vi "Split Numbers.vi"(0 "(hi.lo)":u16) -> (1 "low":u8, 2 "hi":u8)   [LabVIEW 2010]
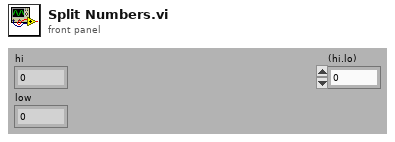
[diagram p1: front panel]
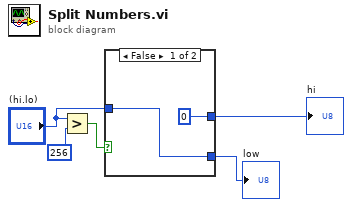
[diagram p0: block diagram]
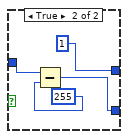
[diagram p2: hidden frame]
diagram:
  n1 = Greater?(x="(hi.lo)", y=u16 256) -> (0:w4:bool)
  n2 = case shown="False" w4 {
    tunnel: [u8 0 ("hi") u8 1 ("hi")] -> w3
    tunnel: "(hi.lo)" -> [w6 w9]
    tunnel: [w6 w8] -> w1
    frame False {
    }
    frame True {
      n3 = Subtract(x=w9, y=u8 255 ("low 2")) -> (x-y=w8:u16)
    }
  }
  "hi" <- w3
  "low" <- w1
